vi "Append VI History to Report (refnum).vi"(0 "report in":refnum<class "NI_report.lvclass">, 5 "VI":refnum<vi>, 11 "error in (no error)":errorcluster, 12 "MS Office parameters":T1) -> (4 "report out":refnum<class "NI_report.lvclass">, 6 "VI out":refnum<vi>, 8 "start out (Word)":i32, 10 "end out (Word)":i32, 15 "error out":errorcluster)   [LabVIEW 2017, in "NI_ReportGenerationCore.lvlib"]
doc: "Appends the revision history of the VI you specify in <B>VI</B> to a report. Wire data to the <B>VI</B> input to determine the polymorphic instance to use or manually select the instance."
uses:
  <vilib>/Utility/NIReport.llb/NI_ReportGenerationCore.lvlib
  <vilib>/Utility/NIReport.llb/NI_report.lvclass
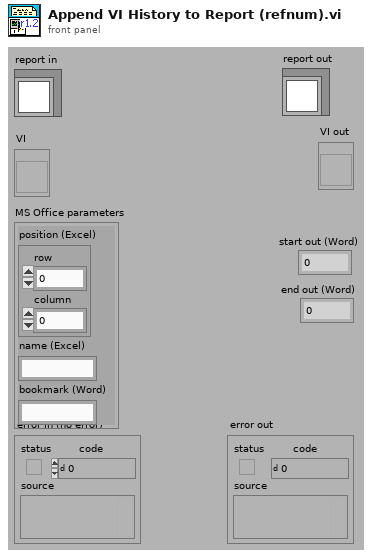
[diagram p1: front panel]
types:
  T1 = cluster{"position (Excel)":cluster{"row":i32, "column":i32}, "name (Excel)":string, "bookmark (Word)":string}
  T2 = enum32{"invalid app kind", "Development System", "Run Time System", "Student Edition", "Embedded LabVIEW", "Evaluation", "Custom"}
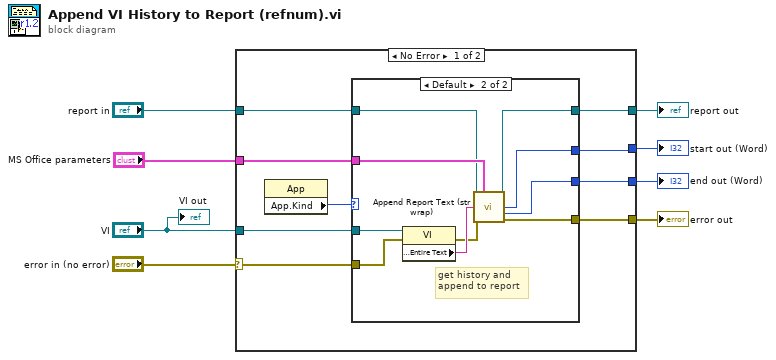
[diagram p0: block diagram]
diagram:
  n1 = case shown="No Error" "error in (no error)" {
    selector: "error in (no error)" -> [w16 w31]
    tunnel: [w14 w31] -> w7
    tunnel: [w11 w30] -> w5
    tunnel: "report in" -> [w10 w30]
    tunnel: "VI" -> [w17 _]
    tunnel: "MS Office parameters" -> [w15 _]
    tunnel: [w13 _] -> w2
    tunnel: [w12 _] -> w1
    frame No Error {
      n2 = property class="App"() -> ("App.Kind"=w9:T2)  [unwired: 2 in, 2 out]
      n3 = case shown="Default" w9 {
        tunnel: w17 -> [_ w29]
        tunnel: w16 -> [w18 w28]
        tunnel: w15 -> [_ w27]
        tunnel: [w18 w25] -> w14
        tunnel: [_ w23] -> w13
        tunnel: [_ w22] -> w12
        tunnel: [w19 w21] -> w11
        tunnel: w10 -> [w19 w20]
        frame "Run Time System" {
          # "Do not try to append\nif running in an\nexecutable"
        }
        frame Default {
          # "get history and\nappend to report"
          n4 = property class="VI"(reference=w29, error in=w28) -> (error out=w24:errorcluster, "History:Entire Text"=w26:string)  [unwired: 1 out]
          n5 = call <vilib>:"Append Report Text (str wrap).vi"("report in"=w20, "MS Office parameters"=w27, "text"=w26, "error in (no error)"=w24) -> ("report out"=w21:refnum<class "NI_report.lvclass">, "start out (Word)"=w23:i32, "end out (Word)"=w22:i32, "error out"=w25:errorcluster)  [unwired: 8 in]
        }
      }
    }
    frame Error {
    }
  }
  "error out" <- w7
  "report out" <- w5
  "start out (Word)" <- w2
  "end out (Word)" <- w1
  "VI out" <- "VI"
